vi "Final.vi"() -> ()   [LabVIEW 2020]
uses:
  <vilib>/Instr/_visa.llb/VISA Configure Serial Port (Instr).vi
panel:
  in  "VISA resource name":refnum<visa-resource-name>="COM5"
  out "read buffer":string
  in  "stop":bool
  in  "Tab Control":enum32{"Flujo", "Volúmen", "Presión"}(tab)
  out "Flujo":dbl(graph)
  out "Volúmen 2":i32(graph)
  out "Presión 2":dbl(graph)
  out "Waveform Graph":dbl[](graph)
  out "XY Graph":cluster{"X":dbl, "Y":dbl}[](graph)
  out "Frecuencia":ext format="%#.1p"
  out "Operación":string
  out "Pausa [s]":dbl format="%#.1g"
  out "Relación":dbl format="%#.1g"
  out "T_Expiración [s]":dbl format="%#.1g"
  out "FIO2 [%]":u8
  out "Estado":string
  out "T_Inspiración [s]":dbl format="%#.1g"
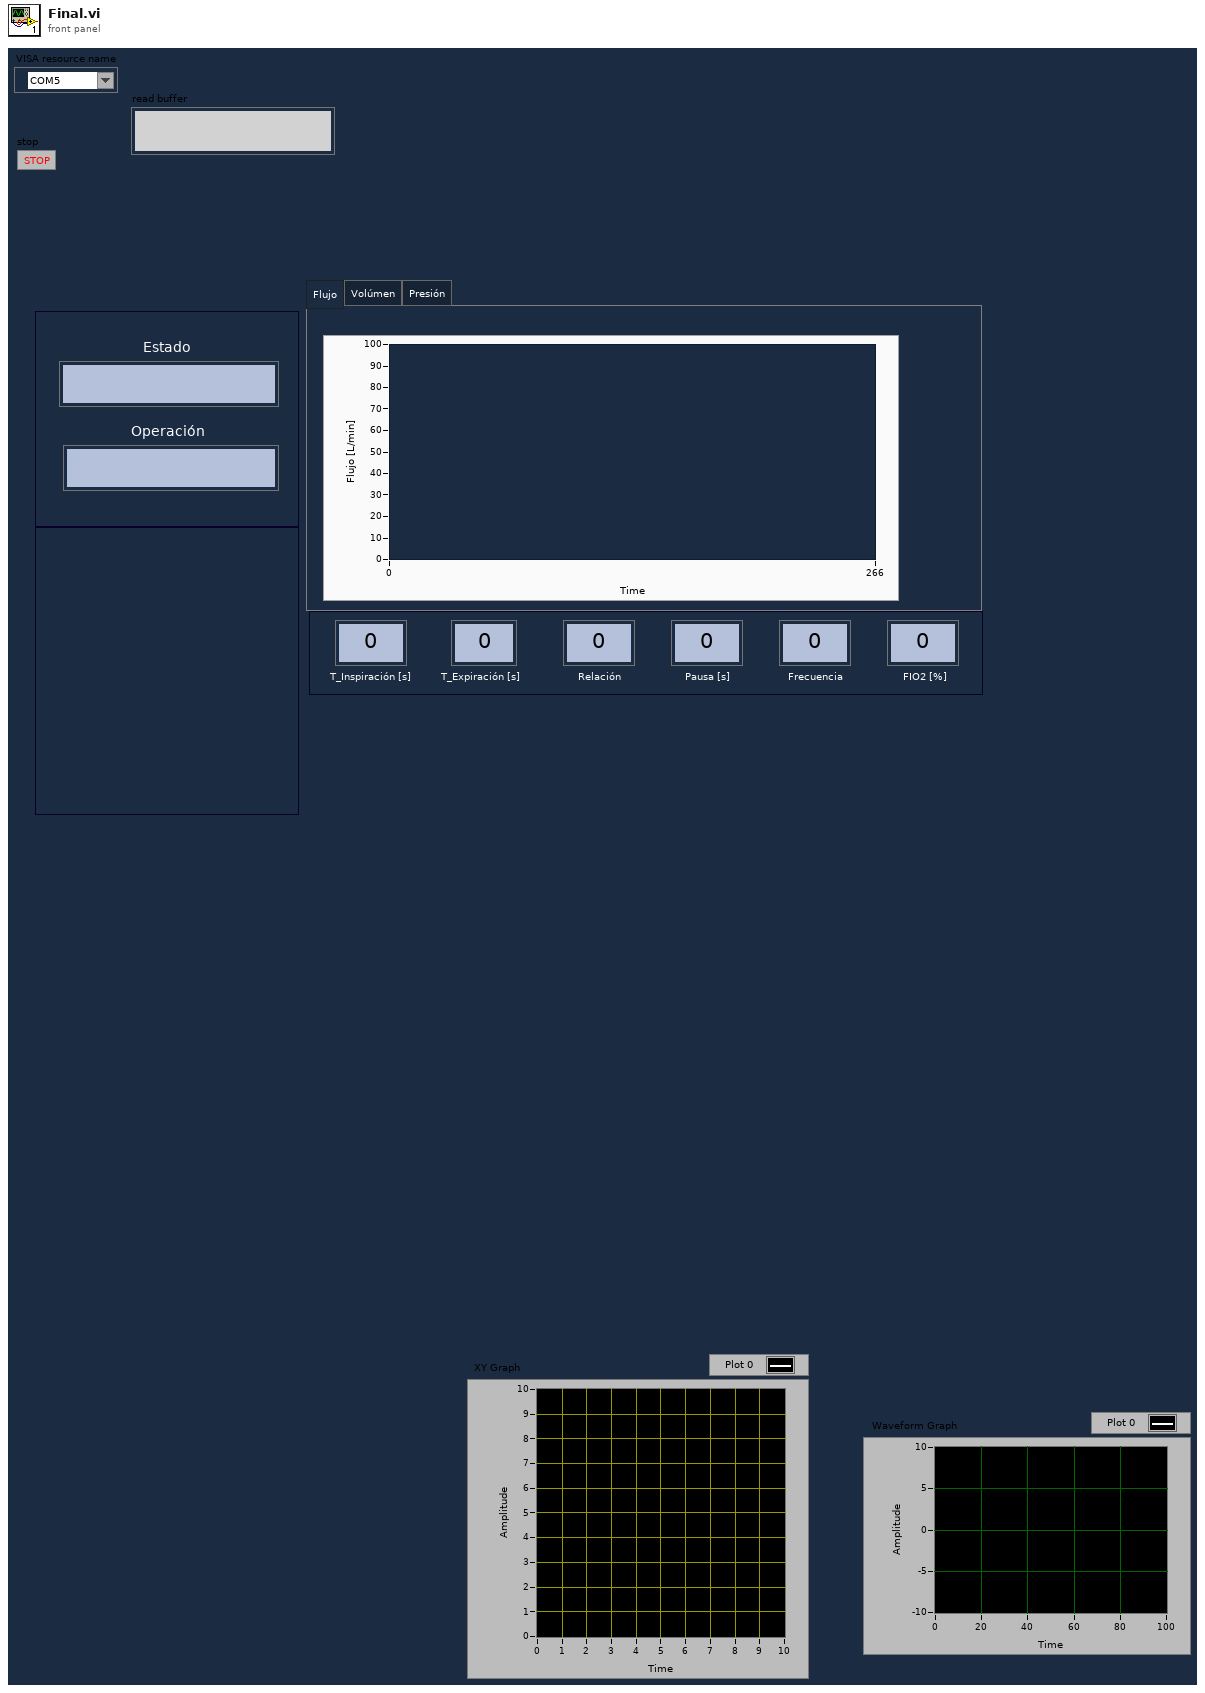
[diagram p1: front panel]
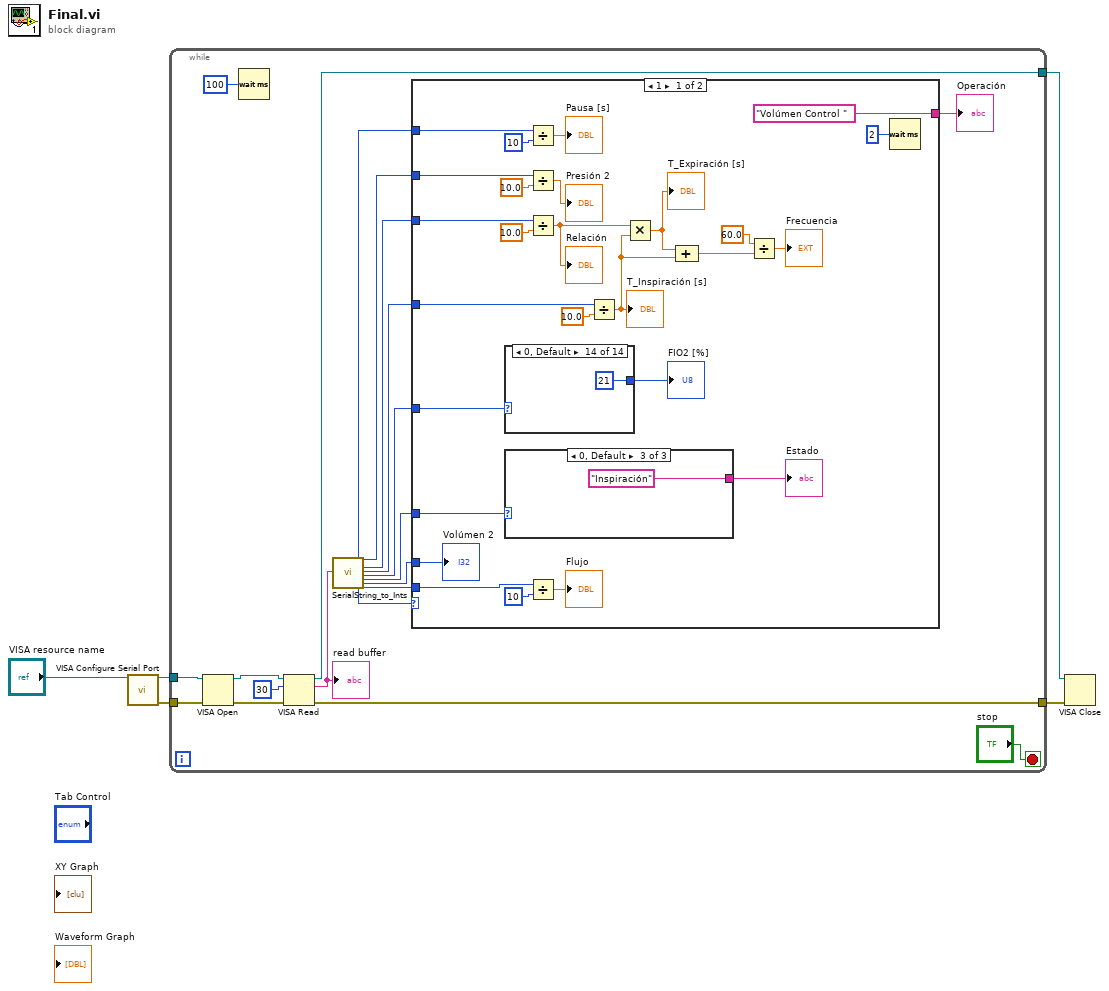
[diagram p0: block diagram]
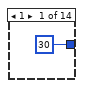
[diagram p2: hidden frame]
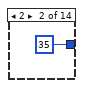
[diagram p3: hidden frame]
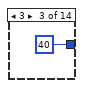
[diagram p4: hidden frame]
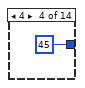
[diagram p5: hidden frame]
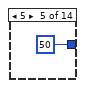
[diagram p6: hidden frame]
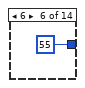
[diagram p7: hidden frame]
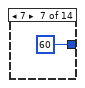
[diagram p8: hidden frame]
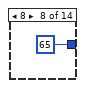
[diagram p9: hidden frame]
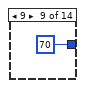
[diagram p10: hidden frame]
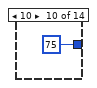
[diagram p11: hidden frame]
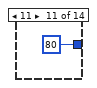
[diagram p12: hidden frame]
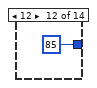
[diagram p13: hidden frame]
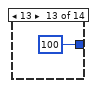
[diagram p14: hidden frame]
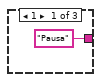
[diagram p15: hidden frame]
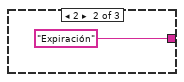
[diagram p16: hidden frame]
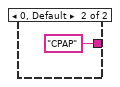
[diagram p17: hidden frame]
diagram:
  n1 = call-poly "VISA Configure Serial Port"("VISA resource name"="VISA resource name") -> ("VISA resource name out"=w3:refnum<visa-resource-name>, "error out"=w2:errorcluster)  [unwired: 13 in]
  n2 = while {
    tunnel: [w25] -> w5
    tunnel: w2 -> [w23]
    tunnel: w3 -> [w22]
    tunnel: [w20] -> w4
    stop <- "stop" stop-if-true
    n3 = VISA Open(error in (no error)=w23, VISA resource name=w22) -> (VISA resource name=w21:refnum<visa-resource-name>, error out=w24:errorcluster)  [unwired: 3 in]
    n4 = Wait (ms)(milliseconds to wait=u32 100) -> ()  [unwired: 1 out]
    n5 = VISA Read(VISA resource name=w21, byte count=u32 30, error in (no error)=w24) -> (VISA resource name out=w20:refnum<visa-resource-name>, read buffer=w15:string, error out=w25:errorcluster)  [unwired: 1 out]
    "read buffer" <- w15
    n6 = call "SerialString_to_Ints.vi"("input string"=w15) -> ("output 9"=w12:i32, "output 10"=w13:i32, "output 1"=w14:i32, "output 3"=w6:i32, "output 4"=w7:i32, "output 5"=w8:i32, "output 6"=w9:i32, "output 7"=w10:i32, "output 8"=w11:i32)  [unwired: 17 in, 1 out]
    n7 = case shown="1" w13 {
      tunnel: ["Volúmen Control " "CPAP"] -> w16
      tunnel: w9 -> [w33 _]
      tunnel: w12 -> [w32 _]
      tunnel: w10 -> [w31 _]
      tunnel: w11 -> [w30 _]
      tunnel: w8 -> [w29 _]
      tunnel: w6 -> [w28 _]
      tunnel: w14 -> [w27 _]
      tunnel: w7 -> [w26 _]
      frame 1 {
        n8 = case shown="0, Default" w29 {
          tunnel: [30 35 40 45 50 55 60 65 70 75 80 85 100 21] -> w50
          frame 1 {
          }
          frame 2 {
          }
          frame 3 {
          }
          frame 4 {
          }
          frame 5 {
          }
          frame 6 {
          }
          frame 7 {
          }
          frame 8 {
          }
          frame 9 {
          }
          frame 10 {
          }
          frame 11 {
          }
          frame 12 {
          }
          frame 13 {
          }
          frame 0, Default {
          }
        }
        "FIO2 [%]" <- w50
        n9 = case shown="0, Default" w33 {
          tunnel: ["Pausa" "Expiración" "Inspiración"] -> w49
          frame 1 {
          }
          frame 2 {
          }
          frame 0, Default {
          }
        }
        "Estado" <- w49
        n10 = Divide(x=w32, y=u8 10) -> (x/y=→"Pausa [s]":dbl)
        n11 = Divide(x=w27, y=10.0) -> (x/y=→"Presión 2":dbl)
        n12 = Divide(x=w28, y=10.0) -> (x/y=w43:dbl)
        "Relación" <- w43
        n13 = Divide(x=w30, y=u8 10) -> (x/y=→"Flujo":dbl)
        n14 = Divide(x=w26, y=10.0) -> (x/y=w37:dbl)
        "T_Inspiración [s]" <- w37
        n15 = Multiply(x=w43, y=w37) -> (x*y=w38:dbl)
        "T_Expiración [s]" <- w38
        n16 = Compound Arithmetic op=ADD(w38, w37) -> (w40:dbl)
        n17 = Divide(x=60.0, y=w40) -> (x/y=→"Frecuencia":dbl)
        n18 = Wait (ms)(milliseconds to wait=u32 2) -> ()  [unwired: 1 out]
        "Volúmen 2" <- w31
      }
      frame 0, Default {
      }
    }
    "Operación" <- w16
  }
  n19 = VISA Close(VISA resource name=w4, error in (no error)=w5) -> ()  [unwired: 1 out]
